vi "pracownia_6_maska.vi"() -> ()   [LabVIEW 2019]
uses:
  Pracowania_6_global.vi
panel:
  in  "Maska":bool[](array[boolean])
  out "Liczba maskowana":bool[](array[boolean])
  out "Liczba niemaskowana":bool[](array[boolean])
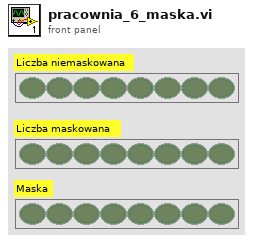
[diagram p1: front panel]
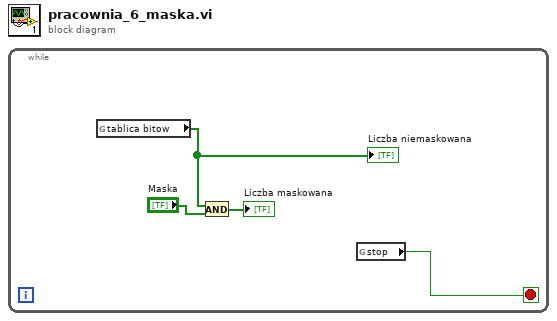
[diagram p0: block diagram]
diagram:
  n1 = while {
    stop <- w1 stop-if-true
    n2 = global read "Pracowania_6_global.vi" "tablica bitow"() -> (w2:bool[])
    "Liczba niemaskowana" <- w2
    n3 = And(x=w2, y="Maska") -> (x .and. y?=→"Liczba maskowana":bool[])
    n4 = global read "Pracowania_6_global.vi" "stop"() -> (w1:bool)
  }
